vi "Drive SS Implem 2016.vi"(10 "Robot Commands":T3, 11 "Drive/Climb State":T1) -> (2 "Drive Actuator Values Out":T2)   [LabVIEW 2015]
uses:
  Robot Commands 2016.ctl
  Load SS/Roller State.ctl
  Drive Actuator Values Out.ctl
  Drive Subsystem State.ctl
  Global Variables/Temp Variables.vi
  Global Variables/Settings.vi
  Global Variables/Calibrations.vi
panel:
  out "Left Motor Drive Speed":dbl(graph)
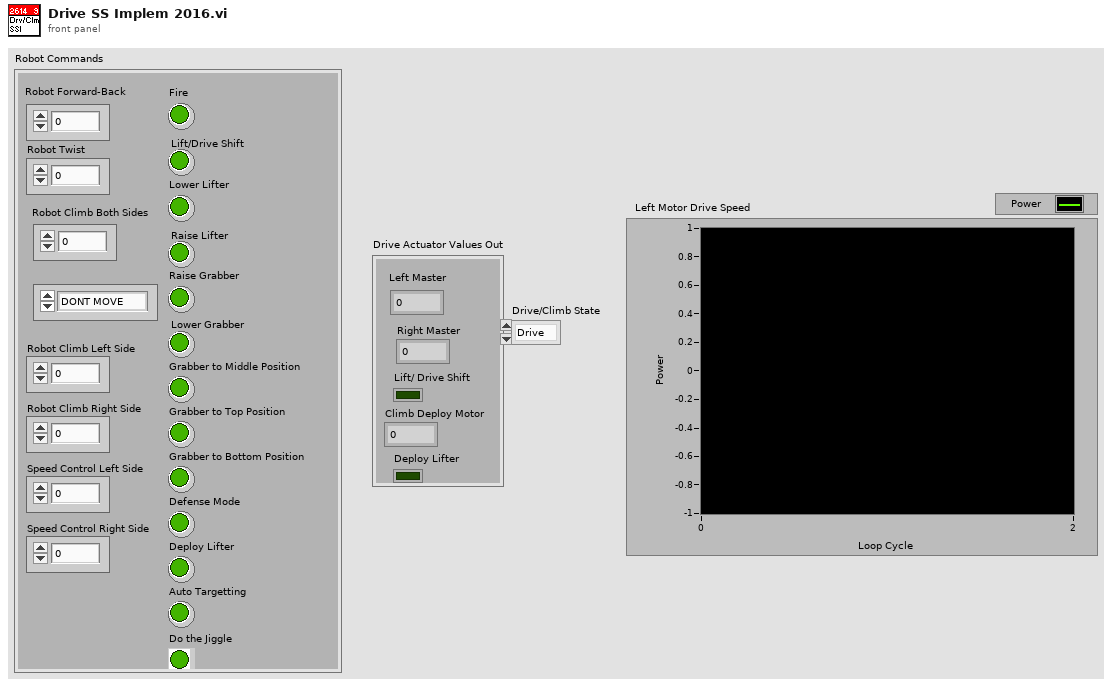
[diagram p1: front panel]
types:
  T1 = typedef "Drive Subsystem State.ctl" = enum16{"Drive", "Climb", "Auto Target"}
  T2 = typedef "Drive Actuator Values Out.ctl" = cluster{"Left Master":dbl, "Right Master":dbl, "Lift/ Drive Shift":bool, "Climb Deploy Motor":dbl, "Deploy Lifter":bool}
  T3 = typedef "Robot Commands 2016.ctl" = cluster{"Robot Forward-Back":dbl, "Robot Twist":dbl, "Fire":bool, "Lift/Drive Shift":bool, "Raise Lifter":bool, "Raise Grabber":bool, "Lower Grabber":bool, "Roller":T4, "Robot Climb Both Sides":dbl, "Grabber to Middle Position":bool, "Grabber to Top Position":bool, "Grabber to Bottom Position":bool, "Robot Climb Left Side":dbl, "Robot Climb Right Side":dbl, "Speed Control Left Side":dbl, "Speed Control Right Side":dbl, "Lower Lifter":bool, "Defense Mode":bool, "Deploy Lifter":bool, "Auto Targetting":bool, "Do the Jiggle":bool}
  T4 = typedef "Roller State.ctl" = enum16{"DONT MOVE", "Intake", "Outtake"}
  T5 = typedef "WPI_CANTalonSRX_APIControlMode.ctl" = enum8{"Percent VBus", "Speed", "Position", "Slave", "Unchanged / Invalid", "Voltage Compensation", "Current", "Motion Profile"}
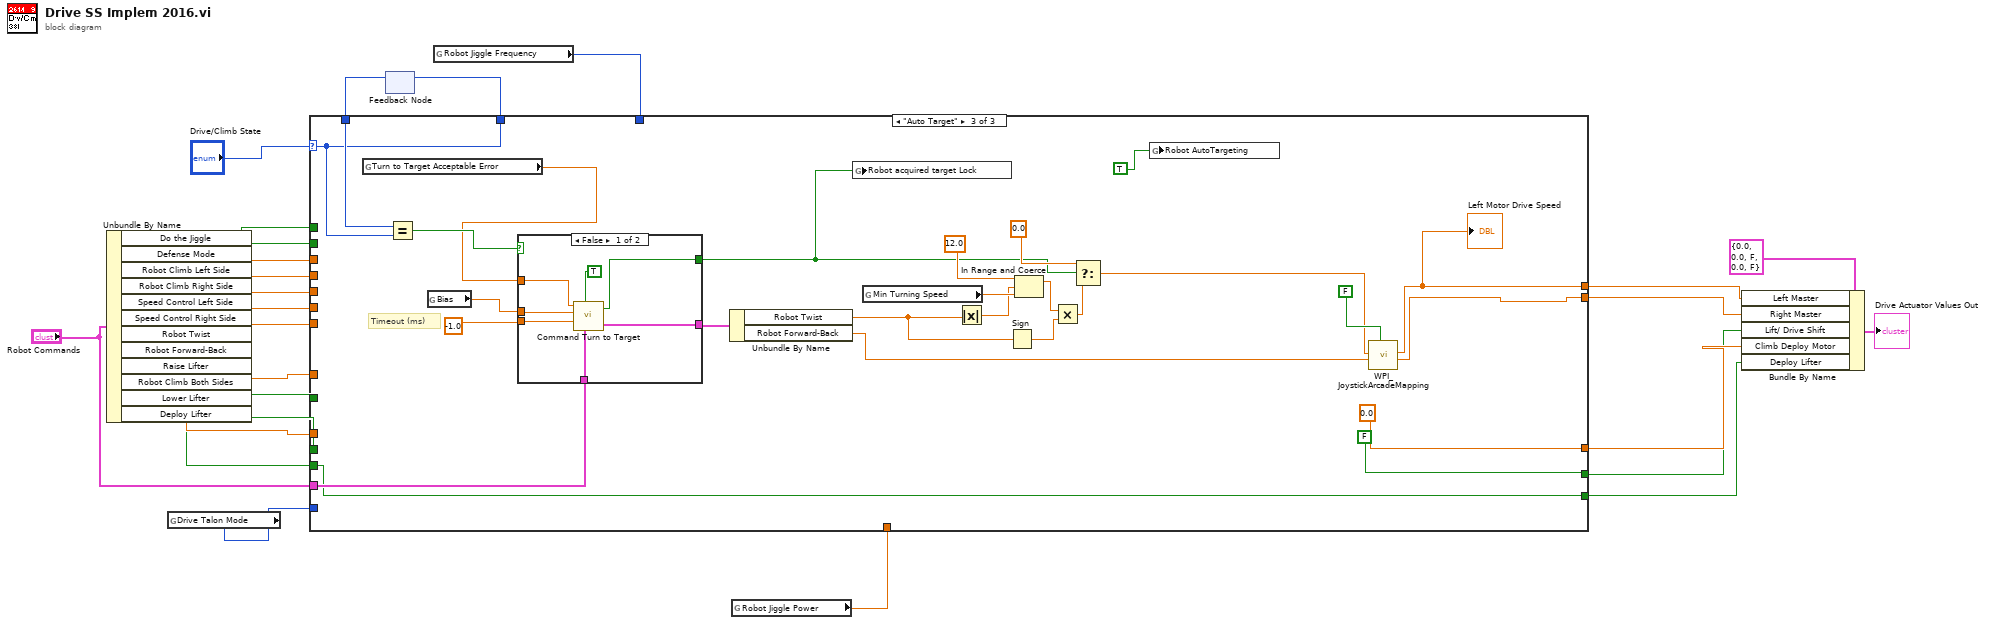
[diagram p0: block diagram]
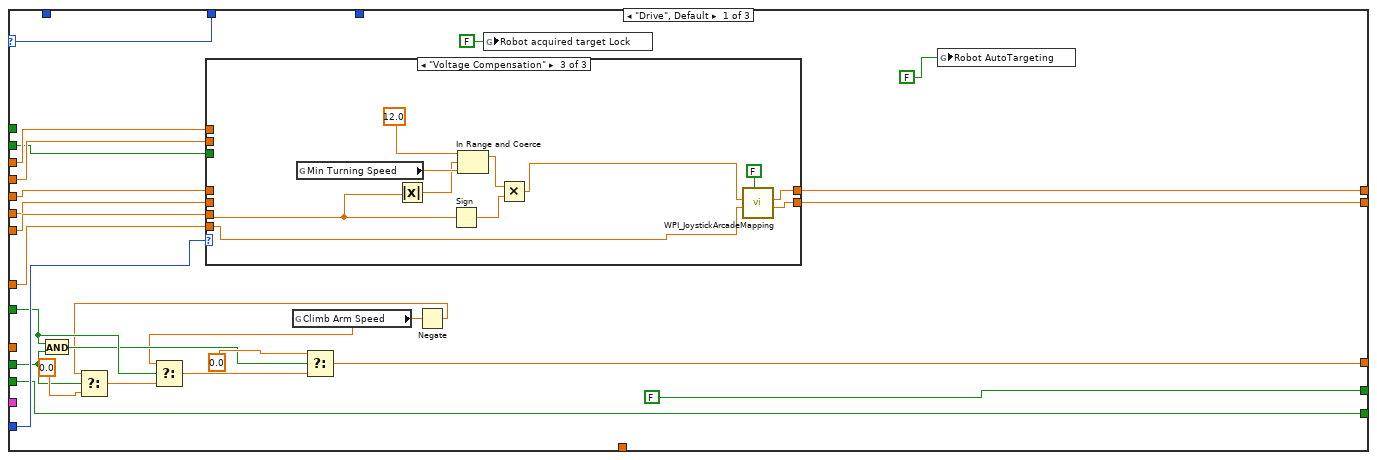
[diagram p2: hidden frame]
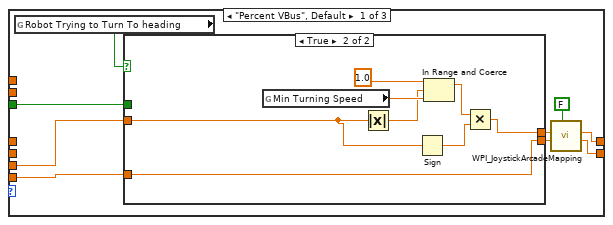
[diagram p3: hidden frame]
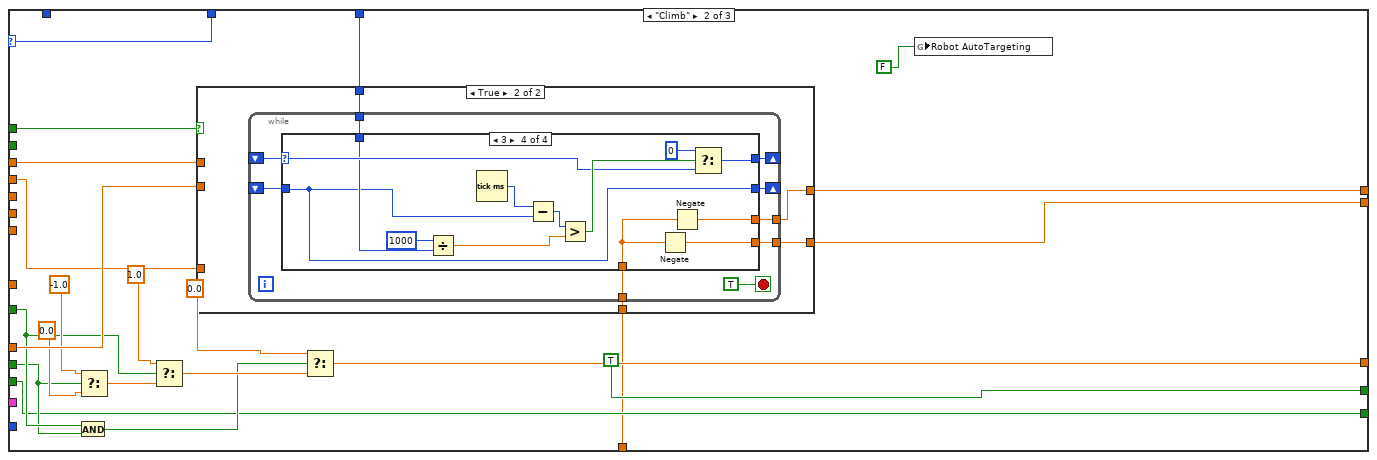
[diagram p6: hidden frame]
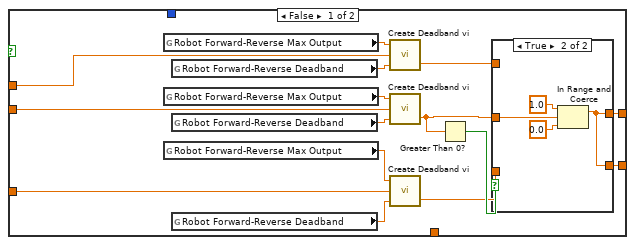
[diagram p7: hidden frame]
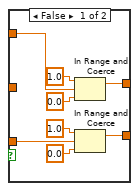
[diagram p8: hidden frame]
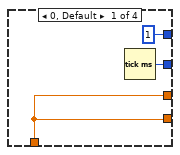
[diagram p9: hidden frame]
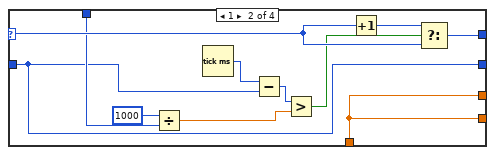
[diagram p10: hidden frame]
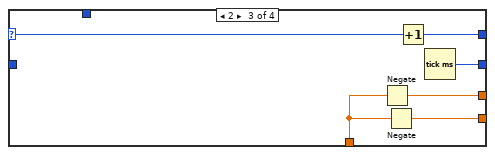
[diagram p11: hidden frame]
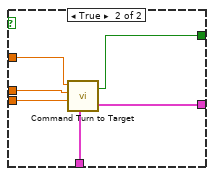
[diagram p12: hidden frame]
diagram:
  n1 = Unbundle By Name("Robot Commands") -> ("Do the Jiggle"=w5:bool, "Defense Mode"=w13:bool, "Robot Climb Left Side"=w19:dbl, "Robot Climb Right Side"=w18:dbl, "Speed Control Left Side"=w17:dbl, "Speed Control Right Side"=w16:dbl, "Robot Twist"=w24:dbl, "Robot Forward-Back"=w23:dbl, "Raise Lifter"=w12:bool, "Robot Climb Both Sides"=w10:dbl, "Lower Lifter"=w15:bool, "Deploy Lifter"=w9:bool)
  n2 = global read "Temp Variables.vi" "Drive Talon Mode"() -> (w21:T5)
  n3 = feedback #1() -> (w6:T1)  [unwired: 1 in]
  n4 = global read "Settings.vi" "Robot Jiggle Frequency"() -> (w4:i32)
  n5 = global read "Settings.vi" "Robot Jiggle Power"() -> (w3:dbl)
  n6 = case shown="\"Auto Target\"" "Drive/Climb State" {
    selector: "Drive/Climb State" -> [w31 w88 w198]
    tunnel: w24 -> [w51 _ _]
    tunnel: w23 -> [w50 _ _]
    tunnel: [w49 w103 w182] -> w1
    tunnel: [w48 w102 w193] -> w20
    tunnel: [FALSE TRUE FALSE ("Startup")] -> w11
    tunnel: w12 -> [w39 w92 _]
    tunnel: [w33 w91 0.0 ("Cmd Parameter 3")] -> w22
    tunnel: w10 -> [_ w104 _]
    tunnel: w21 -> [w46 _ _]
    tunnel: w19 -> [w44 w101 _]
    tunnel: w18 -> [w45 w100 _]
    tunnel: w17 -> [w36 _ _]
    tunnel: w16 -> [w35 _ _]
    tunnel: w15 -> [w38 w90 _]
    tunnel: w13 -> [w34 _ _]
    tunnel: [w32 w89 w195] -> w2
    tunnel: w9 -> [w32 w89 w195]
    tunnel: "Robot Commands" -> [_ _ w201]
    tunnel: [w31 w88 w198] -> w7
    tunnel: w6 -> [_ _ w199]
    tunnel: w5 -> [_ w87 _]
    tunnel: w4 -> [_ w86 _]
    tunnel: w3 -> [_ w85 _]
    frame "Drive", Default {
      n7 = And(x=w39, y=w38) -> (x .and. y?=w37:bool)
      n8 = case shown="\"Voltage Compensation\"" w46 {
        tunnel: w51 -> [w58 _ w73]
        tunnel: w50 -> [w56 _ w74]
        tunnel: [w60 w72 w82] -> w49
        tunnel: [w59 w71 w81] -> w48
        tunnel: w45 -> [_ _ _]
        tunnel: w44 -> [_ _ _]
        tunnel: w36 -> [_ w72 _]
        tunnel: w35 -> [_ w71 _]
        tunnel: w34 -> [w54 _ _]
        frame "Percent VBus", Default {
          n9 = global read "Temp Variables.vi" "Robot Trying to Turn To heading"() -> (w53:bool)
          n10 = case shown="True" w53 {
            tunnel: w58 -> [w62 w63]
            tunnel: [w62 w65] -> w57
            tunnel: w56 -> [w61 w64]
            tunnel: [w61 w64] -> w55
            tunnel: w54 -> [_ _]
            frame False {
            }
            frame True {
              n11 = global read "Settings.vi" "Min Turning Speed"() -> (w69:dbl)
              n12 = Absolute Value(x=w63) -> (abs(x)=w68:dbl)
              n13 = Sign(1:w63) -> (0:w67:dbl)
              n14 = In Range and Coerce(upper limit=1.0 ("y"), x=w68, lower limit=w69) -> (coerced(x)=w66:dbl)  [unwired: 1 out]
              n15 = Multiply(x=w66, y=w67) -> (x*y=w65:dbl)
            }
          }
          n16 = call <vilib>:"WPI_JoystickArcadeMapping.vi"("Square Inputs"=FALSE, "Y axis value"=w55, "X axis value"=w57) -> ("Right Motor Value"=w59:dbl, "Left Motor Value"=w60:dbl)  [unwired: 7 in]
        }
        frame "Speed" {
        }
        frame "Voltage Compensation" {
          n17 = global read "Settings.vi" "Min Turning Speed"() -> (w79:dbl)
          n18 = Absolute Value(x=w73) -> (abs(x)=w78:dbl)
          n19 = Sign(1:w73) -> (0:w77:dbl)
          n20 = In Range and Coerce(upper limit=12.0 ("y"), x=w78, lower limit=w79) -> (coerced(x)=w76:dbl)  [unwired: 1 out]
          n21 = Multiply(x=w76, y=w77) -> (x*y=w75:dbl)
          n22 = call <vilib>:"WPI_JoystickArcadeMapping.vi"("Square Inputs"=FALSE, "Y axis value"=w74, "X axis value"=w75) -> ("Right Motor Value"=w81:dbl, "Left Motor Value"=w82:dbl)  [unwired: 7 in]
        }
      }
      n23 = global read "Calibrations.vi" "Climb Arm Speed"() -> (w28:dbl)
      n24 = Negate(x=w28) -> (-x=w29:dbl)
      n25 = Select(t=w29, s=w38, f=0.0) -> (s? t:f=w42:dbl)
      n26 = Select(t=w28, s=w39, f=w42) -> (s? t:f=w41:dbl)
      n27 = Select(t=0.0, s=w37, f=w41) -> (s? t:f=w33:dbl)
      n28 = global write "Temp Variables.vi" "Robot acquired target Lock"(FALSE ("Robot acquired target Lock")) -> ()
      n29 = global write "Temp Variables.vi" "Robot AutoTargeting"(FALSE ("Robot AutoTargeting")) -> ()
    }
    frame "Climb" {
      n30 = And(x=w92, y=w90) -> (x .and. y?=w93:bool)
      n31 = Select(t=-1.0, s=w90, f=0.0) -> (s? t:f=w97:dbl)
      n32 = Select(t=1.0, s=w92, f=w97) -> (s? t:f=w95:dbl)
      n33 = case shown="True" w87 {
        tunnel: w104 -> [w118 _]
        tunnel: [w110 w136] -> w103
        tunnel: [w109 w135] -> w102
        tunnel: w101 -> [w108 _]
        tunnel: w100 -> [w107 _]
        tunnel: w86 -> [_ w134]
        tunnel: w85 -> [_ w133]
        frame False {
          n34 = global read "Settings.vi" "Robot Forward-Reverse Max Output"() -> (w115:dbl)
          n35 = global read "Settings.vi" "Robot Forward-Reverse Max Output"() -> (w120:dbl)
          n36 = global read "Settings.vi" "Robot Forward-Reverse Max Output"() -> (w116:dbl)
          n37 = global read "Settings.vi" "Robot Forward-Reverse Deadband"() -> (w114:dbl)
          n38 = global read "Settings.vi" "Robot Forward-Reverse Deadband"() -> (w119:dbl)
          n39 = global read "Settings.vi" "Robot Forward-Reverse Deadband"() -> (w117:dbl)
          n40 = call "Create Deadband vi.vi"("Input Deadband"=w114, "Input"=w108, "Output Upper Limit"=w115) -> ("Output"=w112:dbl)  [unwired: 1 in]
          n41 = call "Create Deadband vi.vi"("Input Deadband"=w119, "Input"=w118, "Output Upper Limit"=w120) -> ("Output"=w111:dbl)  [unwired: 1 in]
          n42 = call "Create Deadband vi.vi"("Input Deadband"=w117, "Input"=w107, "Output Upper Limit"=w116) -> ("Output"=w106:dbl)  [unwired: 1 in]
          n43 = Greater Than 0?(x=w111) -> (x > 0?=w113:bool)
          n44 = case shown="True" w113 {
            tunnel: w106 -> [w126 _]
            tunnel: w112 -> [w122 _]
            tunnel: w111 -> [_ w132]
            tunnel: [w121 w131] -> w110
            tunnel: [w125 w131] -> w109
            frame False {
              n45 = In Range and Coerce(upper limit=1.0, x=w122, lower limit=0.0) -> (coerced(x)=w121:dbl)  [unwired: 1 out]
              n46 = In Range and Coerce(upper limit=1.0, x=w126, lower limit=0.0) -> (coerced(x)=w125:dbl)  [unwired: 1 out]
            }
            frame True {
              n47 = In Range and Coerce(upper limit=1.0, x=w132, lower limit=0.0) -> (coerced(x)=w131:dbl)  [unwired: 1 out]
            }
          }
        }
        frame True {
          n48 = while {
            shift-right: [w144] -> _
            shift-left: _ -> [w143]
            shift-right: [w142] -> _
            shift-left: _ -> [w138]
            tunnel: [w141] -> w136
            tunnel: [w140] -> w135
            tunnel: w134 -> [w139]
            tunnel: w133 -> [w137]
            stop <- TRUE stop-if-true
            n49 = case shown="3" w143 {
              selector: w143 -> [_ w158 w165 w173]
              tunnel: [1 w159 w164 w172] -> w144
              tunnel: [w148 w150 w163 w170] -> w142
              tunnel: [w146 w149 w161 w166] -> w141
              tunnel: [w146 w149 w160 w167] -> w140
              tunnel: w139 -> [_ w156 _ w171]
              tunnel: w138 -> [_ w150 _ w170]
              tunnel: w137 -> [w146 w149 w162 w168]
              frame 0, Default {
                n50 = Tick Count (ms)() -> (millisecond timer value=w148:u32)
              }
              frame 1 {
                n51 = Divide(x=1000, y=w156) -> (x/y=w152:dbl)
                n52 = Tick Count (ms)() -> (millisecond timer value=w154:u32)
                n53 = Subtract(x=w154, y=w150) -> (x-y=w153:u32)
                n54 = Greater?(x=w153, y=w152) -> (0:w151:bool)
                n55 = Increment(x=w158) -> (x+1=w157:i32)
                n56 = Select(t=w157, s=w151, f=w158) -> (s? t:f=w159:i32)
              }
              frame 2 {
                n57 = Negate(x=w162) -> (-x=w161:dbl)
                n58 = Negate(x=w162) -> (-x=w160:dbl)
                n59 = Increment(x=w165) -> (x+1=w164:i32)
                n60 = Tick Count (ms)() -> (millisecond timer value=w163:u32)
              }
              frame 3 {
                n61 = Divide(x=1000, y=w171) -> (x/y=w175:dbl)
                n62 = Tick Count (ms)() -> (millisecond timer value=w177:u32)
                n63 = Subtract(x=w177, y=w170) -> (x-y=w176:u32)
                n64 = Greater?(x=w176, y=w175) -> (0:w174:bool)
                n65 = Negate(x=w168) -> (-x=w167:dbl)
                n66 = Negate(x=w168) -> (-x=w166:dbl)
                n67 = Select(t=0, s=w174, f=w173) -> (s? t:f=w172:i32)
              }
            }
          }
        }
      }
      n68 = Select(t=0.0, s=w93, f=w95) -> (s? t:f=w91:dbl)
      n69 = global write "Temp Variables.vi" "Robot AutoTargeting"(FALSE ("Robot AutoTargeting")) -> ()
    }
    frame "Auto Target" {
      # "Timeout (ms)"
      n70 = global read "Settings.vi" "Turn to Target Acceptable Error"() -> (w196:dbl)
      n71 = Equal?(x=w199, y=w198) -> (x = y?=w197:bool)
      n72 = global read "Calibrations.vi" "Bias"() -> (w179:dbl)
      n73 = case shown="False" w197 {
        tunnel: [w208 w217] -> w202
        tunnel: w201 -> [w209 w216]
        tunnel: -1.0 ("Cmd Parameter 3") -> [w211 w215]
        tunnel: w196 -> [w207 w214]
        tunnel: [w206 w213] -> w181
        tunnel: w179 -> [w205 w212]
        frame False {
          n74 = call "Command Turn to Target.vi"("Input Robot Commands"=w209, "Startup"=TRUE, "Cmd Parameter 3"=w211, "Cmd Parameter 2"=w205, "Cmd Parameter 1"=w207) -> ("Output Robot Commands"=w208:T3, "Completed"=w206:bool)  [unwired: 1 in]
        }
        frame True {
          n75 = call "Command Turn to Target.vi"("Input Robot Commands"=w216, "Cmd Parameter 3"=w215, "Cmd Parameter 2"=w212, "Cmd Parameter 1"=w214) -> ("Output Robot Commands"=w217:T3, "Completed"=w213:bool)  [unwired: 2 in]
        }
      }
      n76 = Unbundle By Name(w202) -> ("Robot Twist"=w186:dbl, "Robot Forward-Back"=w192:dbl)
      n77 = global write "Temp Variables.vi" "Robot acquired target Lock"(w181) -> ()
      n78 = global read "Settings.vi" "Min Turning Speed"() -> (w188:dbl)
      n79 = Absolute Value(x=w186) -> (abs(x)=w187:dbl)
      n80 = Sign(1:w186) -> (0:w185:dbl)
      n81 = In Range and Coerce(upper limit=12.0 ("y"), x=w187, lower limit=w188) -> (coerced(x)=w184:dbl)  [unwired: 1 out]
      n82 = Multiply(x=w184, y=w185) -> (x*y=w183:dbl)
      n83 = Select(t=0.0 ("y"), s=w181, f=w183) -> (s? t:f=w189:dbl)
      n84 = global write "Temp Variables.vi" "Robot AutoTargeting"(TRUE ("Robot AutoTargeting")) -> ()
      n85 = call <vilib>:"WPI_JoystickArcadeMapping.vi"("Square Inputs"=FALSE, "Y axis value"=w192, "X axis value"=w189) -> ("Right Motor Value"=w193:dbl, "Left Motor Value"=w182:dbl)  [unwired: 7 in]
      "Left Motor Drive Speed" <- w182
    }
  }
  n86 = feedback-in #1(w7) -> ()
  n87 = Bundle By Name(cluster=T2 {"Left Master"=0.0, "Right Master"=0.0, "Lift/ Drive Shift"=FALSE, "Climb Deploy Motor"=0.0, "Deploy Lifter"=FALSE} ("Drive Actuator Values"), "Left Master"=w1, "Right Master"=w20, "Lift/ Drive Shift"=w11, "Climb Deploy Motor"=w22, "Deploy Lifter"=w2) -> (→"Drive Actuator Values Out":T2)
